vi "Invert Arcade Drive.vi"(8 "Toggle":bool, 10 "Value 2":dbl, 11 "Value 1":dbl) -> (1 "Value 2":dbl, 2 "Value 1":dbl)   [LabVIEW 2015]
uses:
  <vilib>/Rock Robotics/Network Tables/NT Write Boolean.vi
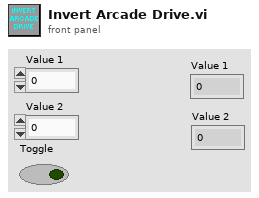
[diagram p1: front panel]
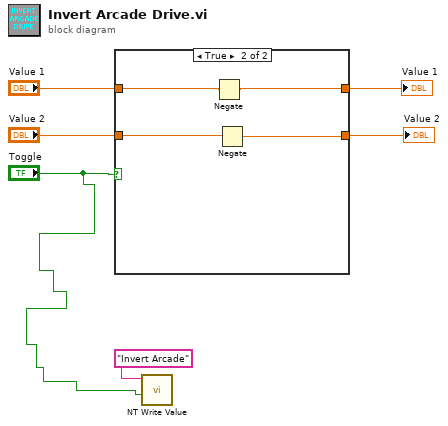
[diagram p0: block diagram]
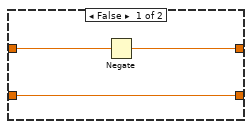
[diagram p2: hidden frame]
diagram:
  n1 = case shown="True" "Toggle" {
    tunnel: "Value 1" -> [w8 w13]
    tunnel: [w7 w12] -> w5
    tunnel: [w9 w10] -> w4
    tunnel: "Value 2" -> [w9 w11]
    frame False {
      n2 = Negate(x=w8) -> (-x=w7:dbl)
    }
    frame True {
      n3 = Negate(x=w13) -> (-x=w12:dbl)
      n4 = Negate(x=w11) -> (-x=w10:dbl)
    }
  }
  "Value 1" <- w5
  "Value 2" <- w4
  n5 = call-poly <vilib>:"NT Write Value.vi"("Boolean"="Toggle", "Name"="Invert Arcade") -> ()  [unwired: 9 in, 1 out]
